vi "SMR_LabVIEW_V7.6.vi"() -> ()   [LabVIEW 2025]
uses:
  <vilib>/DAQmx/write.llb/DAQmx Write (Analog DBL 1Chan 1Samp).vi
  <vilib>/DAQmx/read.llb/DAQmx Read (Analog 1D DBL NChan 1Samp).vi
  <vilib>/DAQmx/read.llb/DAQmx Read (Analog 1D DBL 1Chan NSamp).vi
  <vilib>/Analysis/baseanly.llb/Mean (DBL).vi
  <vilib>/DAQmx/create/channels.llb/DAQmx Create Channel (AI-Temperature-Thermocouple).vi
  <vilib>/DAQmx/create/channels.llb/DAQmx Create Channel (AI-Voltage-Basic).vi
  <vilib>/DAQmx/create/channels.llb/DAQmx Create Channel (AO-Voltage-Basic).vi
  <vilib>/DAQmx/miscellaneous.llb/DAQmx Fill In Error Info.vi
  <vilib>/DAQmx/configure/timing.llb/DAQmx Timing (Sample Clock).vi
  <vilib>/addons/control/pid/pid.llb/PID (DBL).vi
  <vilib>/addons/control/pid/NI_PID_pid.lvlib
  <vilib>/Analysis/NI_AALBase.lvlib
panel:
  out "Voltage Across Rod (V)":dbl format="%0.2f"
  out "Current Run Folder":path
  in  "Log Root Folder":path=path "C:/Users/LocalUser/Documents/GitHub/thermal-loop/resources/v0.1.1/data/001"
  out "Raw NI9201 \nVoltage Display":T1
  in  "Loop Period (ms)":dbl=1000.0
  in  "Stop":bool
  out "Auto Steady State Threshold (deg C/min)":dbl
  out "Max dT/dt (deg C/min)":dbl
  out "Temp Change Rate (deg C/min)":dbl
  out "5-Min Baseline Complete":bool
  out "Rate Window Ready":bool
  out "Steady State":bool
  in  "Voltage Limit (V)":dbl=10.0
  in  "Temperature Limit (C)":dbl=50.0
  in  "Pressure Limit (psi)":dbl=15.0
  out "Max Voltage":bool
  out "Max Temperature":bool
  out "Max Pressure":bool
  out "Heat Exchanger Pressure History":dbl(graph)
  out "Main Loop Pressure History":T2(graph)
  out "Overall Avg Pressure (psi)":dbl
  out "Heat Exchanger Pressure P6 (psi)":dbl
  out "Main Loop Avg Pressure (psi)":dbl
  out "Pressure Display":T3
  out "Overall Pressure History":T4(graph)
  out "Max Loop Pressure (psi)":dbl
  out "Heat Exchanger Temperature History":cluster{"Waveform":dbl, "Waveform":dbl}(graph)
  out "Main Loop Temeperature History":T5(graph)
  out "Heat Exchanger Avg Temp (deg C)":dbl
  out "Temperature Display":T6
  out "Overall Temperature History":T7(graph)
  out "Overall Avg Temp (deg C)":dbl
  out "Max Loop Temp (deg C)":dbl
  out "Final P-Valve Voltage (V)":dbl
  out "PID Trim Voltage (V)":dbl
  in  "PID Temp Setpoint (deg C)":dbl
  in  "Auto PID Enable":bool
  in  "Manual P-Valve Voltage (V)":dbl min=0.0 max=10.0
  out "Main Loop Avg Temp (deg C)":dbl
  out "Flow History":dbl(graph)
  out "Heat Exchanger Flow (GPM)":dbl
  # "Control/Troubleshoot"
  # "Steady State"
  # "Emergency Indicators"
  # "Pressure"
  # "Temperature"
  # "Proportional Valve Control"
  # "Heat Exchanger Flow"
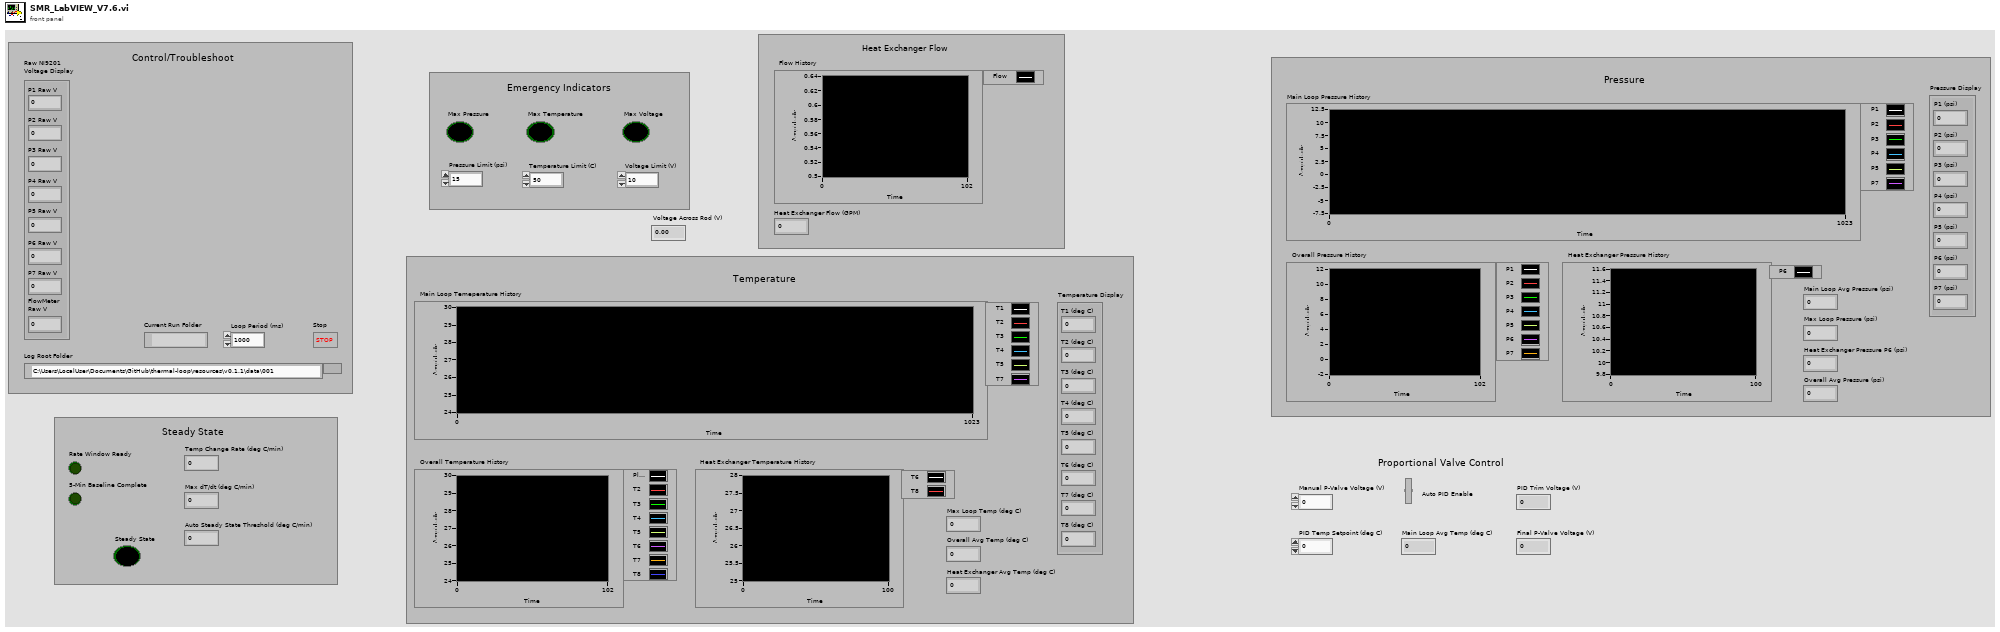
[diagram p1: front panel]
types:
  T1 = cluster{"P1 Raw V":dbl, "P2 Raw V":dbl, "P3 Raw V":dbl, "P4 Raw V":dbl, "P5 Raw V":dbl, "P6 Raw V":dbl, "P7 Raw V":dbl, "FlowMeter\nRaw V":dbl}
  T2 = cluster{"P1":dbl, "P2":dbl, "P3":dbl, "P4":dbl, "P5":dbl, "P7":dbl}
  T3 = cluster{"P1 (psi)":dbl, "P2 (psi)":dbl, "P3 (psi)":dbl, "P4 (psi)":dbl, "P5 (psi)":dbl, "P6 (psi)":dbl, "P7 (psi)":dbl}
  T4 = cluster{"P1":dbl, "P2":dbl, "P3":dbl, "P4":dbl, "P5":dbl, "P6":dbl, "P7":dbl}
  T5 = cluster{"Waveform":dbl, "Waveform":dbl, "Waveform":dbl, "Waveform":dbl, "Waveform":dbl, "Waveform":dbl}
  T6 = cluster{"T1 (deg C)":dbl, "T2 (deg C)":dbl, "T3 (deg C)":dbl, "T4 (deg C)":dbl, "T5 (deg C)":dbl, "T6 (deg C)":dbl, "T7 (deg C)":dbl, "T8 (deg C)":dbl}
  T7 = cluster{"Waveform":dbl, "Waveform":dbl, "Waveform":dbl, "Waveform":dbl, "Waveform":dbl, "Waveform":dbl, "Waveform":dbl, "Waveform":dbl}
  T8 = enum16{"open", "replace", "create", "open or create", "replace or create", "replace or create with confirmation"}
  T9 = cluster{"proportional gain (Kc)":dbl, "integral time (Ti, min)":dbl, "derivative time (Td, min)":dbl}
  T10 = cluster{"P1":dbl, "P2":dbl, "P3":dbl, "P4":dbl, "P5":dbl, "P6":dbl, "P7":dbl, "Flow":dbl}
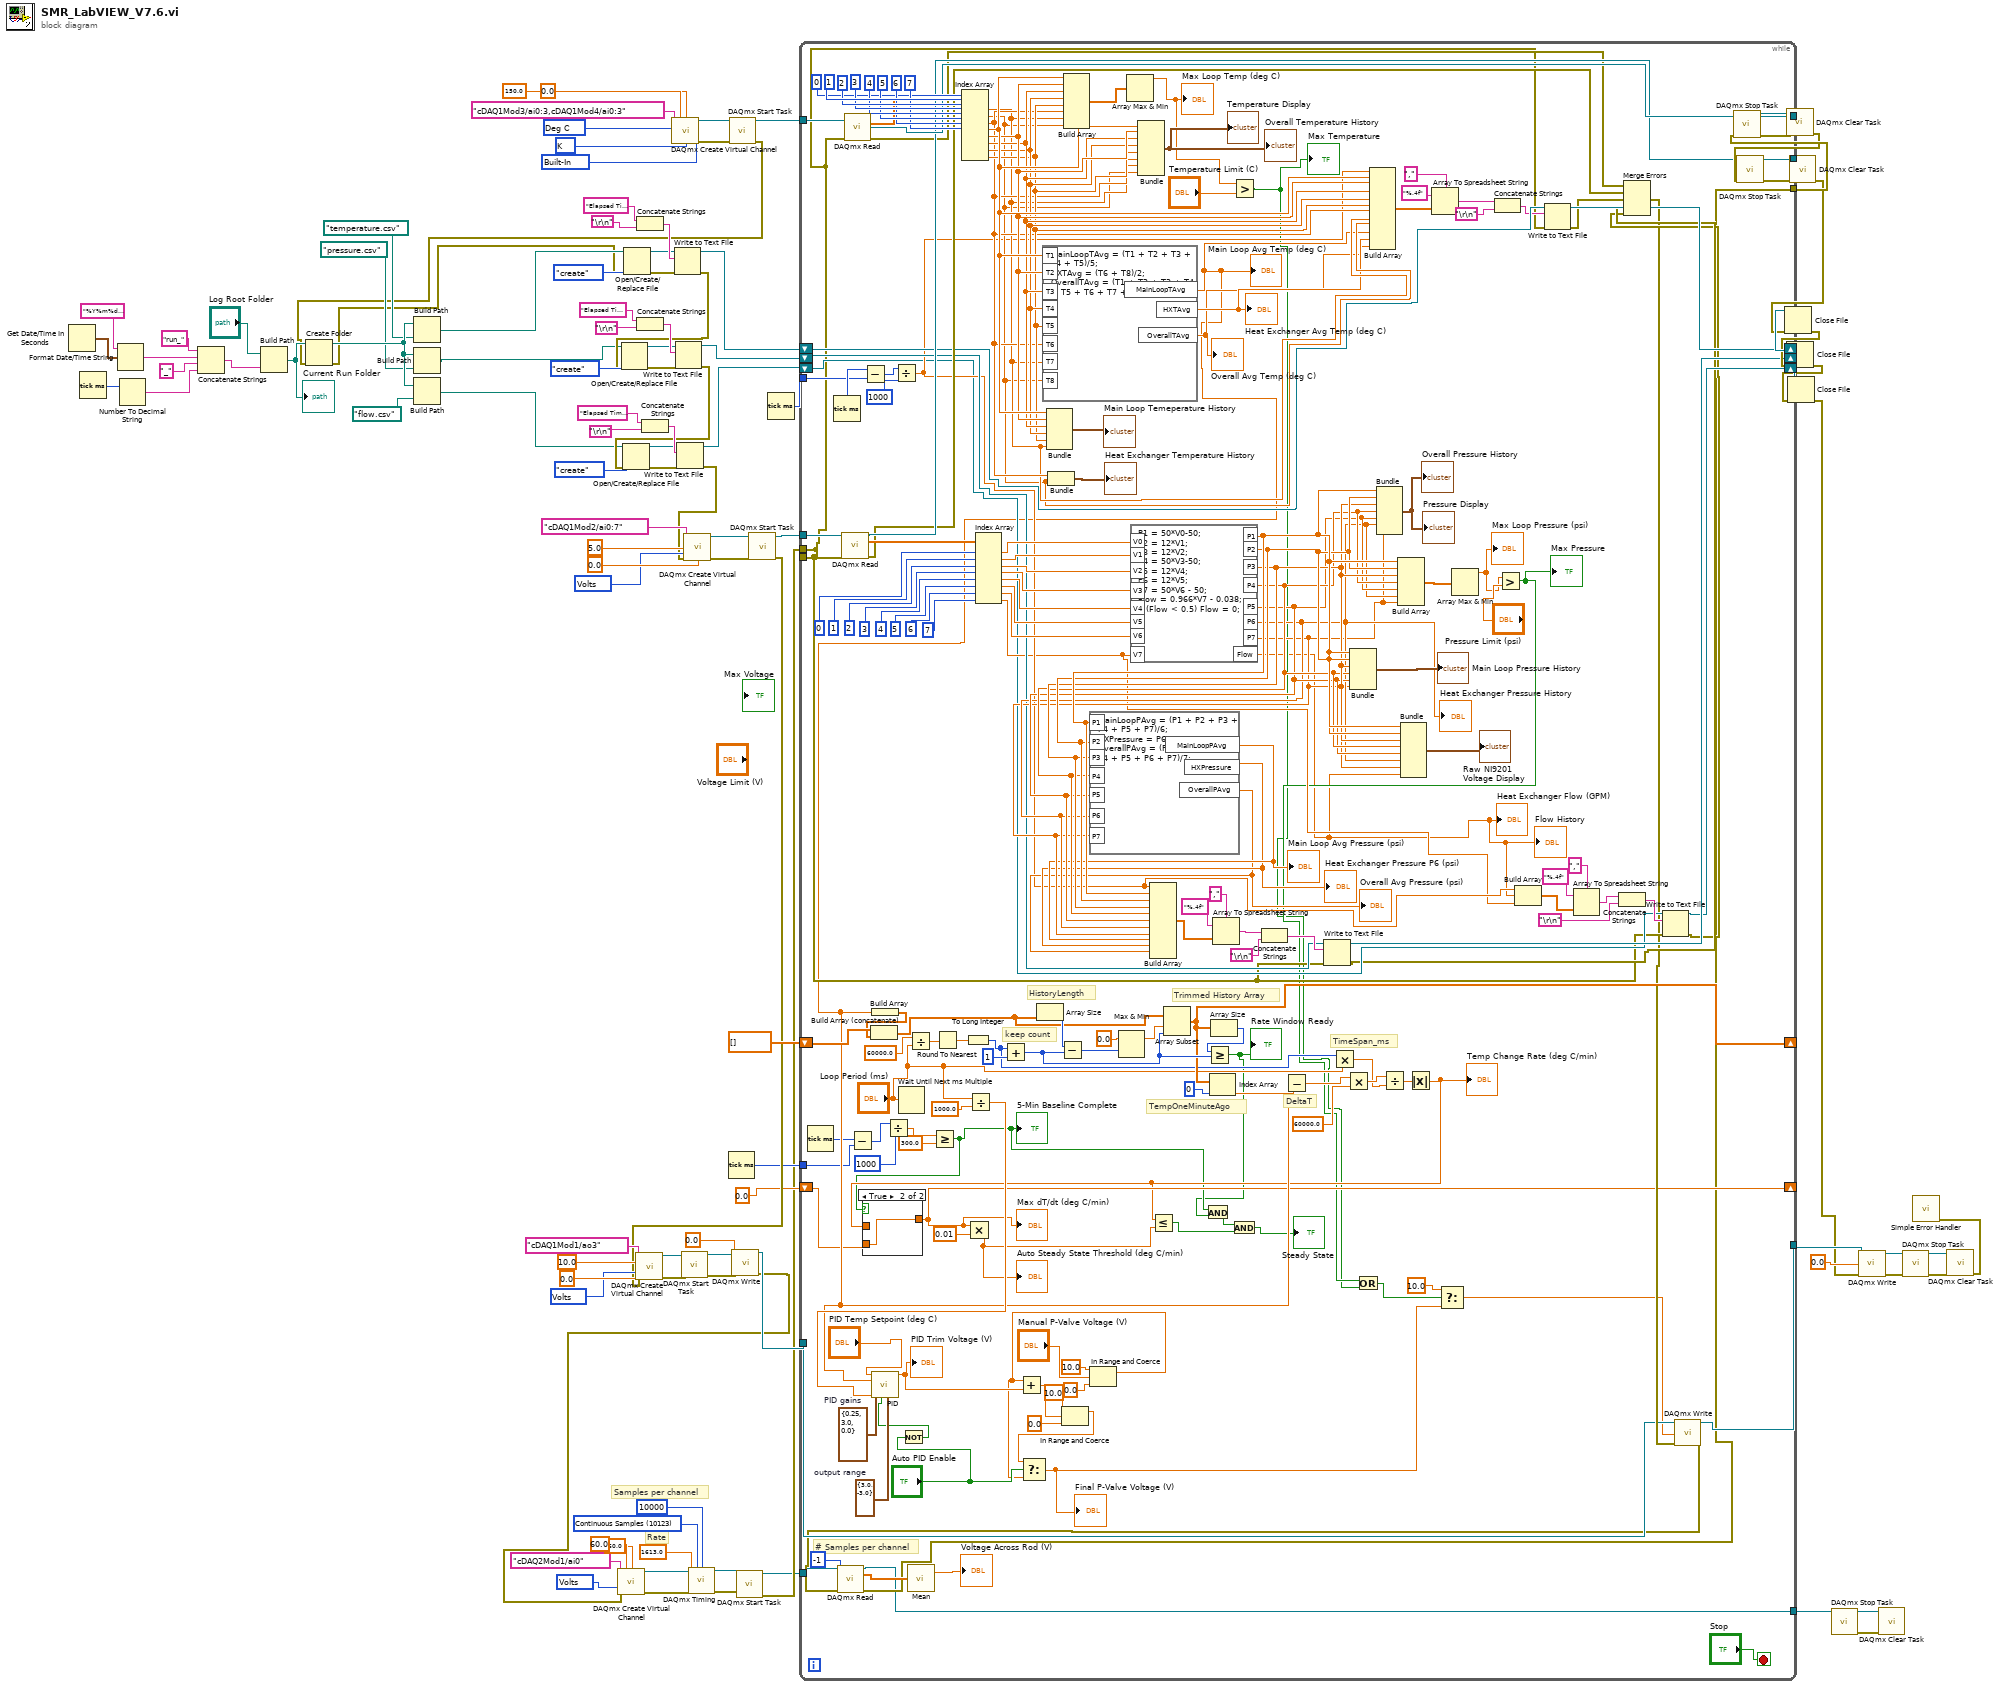
[diagram p0: block diagram]
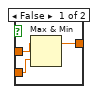
[diagram p2: hidden frame]
diagram:
  w12 = 10123 items=["Finite Samples"=10178, "Continuous Samples"=10123, "Hardware Timed Single Point"=12522] ("sample mode")
  w14 = 10348 items=["Volts"=10348, "From Custom Scale"=10065] ("units")
  w35 = 10348 items=["Volts"=10348, "From Custom Scale"=10065] ("units")
  w101 = 10200 items=["Built-In"=10200, "Constant Value"=10116, "Channel"=10113] ("cjc source")
  w102 = 10073 items=["J"=10072, "K"=10073, "N"=10077, "R"=10082, "S"=10085, "T"=10086, "B"=10047, "E"=10055] ("thermocouple type")
  w103 = 10143 items=["Deg C"=10143, "Deg F"=10144, "Kelvins"=10325, "Deg R"=10145, "From Custom Scale"=10065] ("units")
  w110 = 10348 items=["Volts"=10348, "From Custom Scale"=10065] ("units")
  # "Samples per channel"
  # "Rate"
  n1 = Get Date/Time In Seconds() -> (seconds since 1Jan1904=w58:timestamp)
  n2 = Tick Count (ms)() -> (millisecond timer value=w56:u32)
  n3 = Format Date/Time String(time format string (%c)="%Y%m%d_%H%M%S", seconds (now)=w58) -> (date/time string=w53:string)  [unwired: 1 in]
  n4 = Number To Decimal String(number=w56) -> (decimal integer string=w54:string)  [unwired: 1 in]
  n5 = Concatenate Strings("run_" ("string"), w53, "_" ("string"), w54) -> (w50:string)
  n6 = Build Path(base path="Log Root Folder", name or relative path=w50) -> (appended path=w49:path)
  "Current Run Folder" <- w49
  n7 = Concatenate Strings("Elapsed Time (s),T1 (deg C),T2 (deg C),T3 (deg C),T4 (deg C),T5 (deg C),T6 (deg C),T7 (deg C),T8 (deg C),Main Loop Avg Temp (deg C),HX Avg Temp (deg C),Overall Avg Temp (deg C)", "\r\n") -> (w84:string)
  n8 = Concatenate Strings("Elapsed Time (s),P1 (psi),P2 (psi),P3 (psi),P4 (psi),P5 (psi),P6 (psi),P7 (psi),Main Loop Avg Pressure (psi),HX Pressure (psi),Overall Avg Pressure (psi)", "\r\n") -> (w82:string)
  n9 = Concatenate Strings("Elapsed Time (s),Heat Exchanger Flow (GPM),Flow Raw Voltage (V)", "\r\n") -> (w78:string)
  n10 = call-poly <vilib>:"DAQmx Create Virtual Channel.vi"("maximum value"=150.0, "minimum value"=0.0, "physical channels"=tag "cDAQ1Mod3/ai0:3,cDAQ1Mod4/ai0:3", "cjc source"=w101, "units"=w103, "thermocouple type"=w102) -> ("task out"=w100:refnum<k21>, "error out"=w99:errorcluster)  [unwired: 8 in]
  n11 = Tick Count (ms)() -> (millisecond timer value=w19:u32)
  n12 = call <vilib>:"DAQmx Start Task.vi"("task/channels in"=w100, "error in"=w99) -> ("task out"=w98:refnum<k21>, "error out"=w41:errorcluster)  [unwired: 12 in]
  n13 = Create Folder(path (use dialog)=w49, error in=w41) -> (created path=w48:path, error out=w40:errorcluster)  [unwired: 1 in, 1 out]
  n14 = Build Path(base path=w48, name or relative path=path "temperature.csv") -> (appended path=w47:path)
  n15 = Build Path(base path=w48, name or relative path=path "pressure.csv") -> (appended path=w46:path)
  n16 = Build Path(base path=w48, name or relative path=path "flow.csv") -> (appended path=w45:path)
  n17 = Open/Create/Replace File(file path (use dialog)=w47, error in=w40, operation (0:open)=T8."create") -> (refnum out=w83:refnum<file>, error out=w67:errorcluster)  [unwired: 3 in, 1 out]
  n18 = Write to Text File(file (use dialog)=w83, text=w84, error in=w67) -> (refnum out=w74:refnum<file>, error out=w66:errorcluster)  [unwired: 1 in, 1 out]
  n19 = Open/Create/Replace File(file path (use dialog)=w46, error in=w66, operation (0:open)=T8."create") -> (refnum out=w81:refnum<file>, error out=w65:errorcluster)  [unwired: 3 in, 1 out]
  n20 = Write to Text File(file (use dialog)=w81, text=w82, error in=w65) -> (refnum out=w73:refnum<file>, error out=w64:errorcluster)  [unwired: 1 in, 1 out]
  n21 = Open/Create/Replace File(file path (use dialog)=w45, error in=w64, operation (0:open)=T8."create") -> (refnum out=w77:refnum<file>, error out=w63:errorcluster)  [unwired: 3 in, 1 out]
  n22 = Write to Text File(file (use dialog)=w77, text=w78, error in=w63) -> (refnum out=w72:refnum<file>, error out=w62:errorcluster)  [unwired: 1 in, 1 out]
  n23 = call-poly <vilib>:"DAQmx Create Virtual Channel.vi"("maximum value"=5.0, "minimum value"=0.0, "physical channels"=tag "cDAQ1Mod2/ai0:7", "units"=w110, "error in"=w62) -> ("task out"=w109:refnum<k21>, "error out"=w108:errorcluster)  [unwired: 9 in]
  n24 = call <vilib>:"DAQmx Start Task.vi"("task/channels in"=w109, "error in"=w108) -> ("task out"=w107:refnum<k21>, "error out"=w28:errorcluster)  [unwired: 12 in]
  n25 = call-poly <vilib>:"DAQmx Create Virtual Channel.vi"("maximum value"=10.0, "minimum value"=0.0, "physical channels"=tag "cDAQ1Mod1/ao3", "units"=w35, "error in"=w28) -> ("task out"=w34:refnum<k21>, "error out"=w33:errorcluster)  [unwired: 9 in]
  n26 = call <vilib>:"DAQmx Start Task.vi"("task/channels in"=w34, "error in"=w33) -> ("task out"=w32:refnum<k21>, "error out"=w31:errorcluster)  [unwired: 12 in]
  n27 = call-poly <vilib>:"DAQmx Write.vi"("task/channels in"=w32, "data"=0.0, "error in"=w31) -> ("task out"=w29:refnum<k21>, "error out"=w6:errorcluster)  [unwired: 10 in, 1 out]
  n28 = call-poly <vilib>:"DAQmx Create Virtual Channel.vi"("maximum value"=60.0, "minimum value"=-60.0, "physical channels"=tag "cDAQ2Mod1/ai0", "units"=w14, "error in"=w6) -> ("task out"=w3:refnum<k21>, "error out"=w5:errorcluster)  [unwired: 9 in]
  n29 = call-poly <vilib>:"DAQmx Timing.vi"("task/channels in"=w3, "sample mode"=w12, "samples per channel"=10000, "rate"=1613.0, "error in"=w5) -> ("task out"=w10:refnum<k21>, "error out"=w9:errorcluster)  [unwired: 9 in]
  n30 = call <vilib>:"DAQmx Start Task.vi"("task/channels in"=w10, "error in"=w9) -> ("task out"=w2:refnum<k21>, "error out"=w4:errorcluster)  [unwired: 12 in]
  n31 = Tick Count (ms)() -> (millisecond timer value=w71:u32)
  n32 = while {
    tunnel: w107 -> [w282]
    tunnel: w98 -> [w258]
    tunnel: [w248] -> w97
    tunnel: [w163] -> _
    tunnel: [w247] -> w96
    tunnel: [w117] -> w95
    shift-right: [w224] -> w70
    shift-left: w74 -> [w225]
    shift-right: [w205] -> w69
    shift-left: w73 -> [w206]
    shift-right: [w195] -> w68
    shift-left: w72 -> [w196]
    tunnel: w71 -> [w243]
    shift-right: [w174] -> _
    shift-left: dbl[] [] -> [w187]
    tunnel: w29 -> [w154]
    tunnel: w4 -> [w163]
    tunnel: [w161] -> w26
    tunnel: w19 -> [w143]
    shift-right: [w136] -> _
    shift-left: 0.0 -> [w138]
    tunnel: w2 -> [w116]
    tunnel: [w115] -> w1
    stop <- "Stop" stop-if-true
    w159 = cluster{"output high":dbl, "output low":dbl} {"output high"=3.0, "output low"=-3.0}  # output range
    w160 = T9 {"proportional gain (Kc)"=0.25, "integral time (Ti, min)"=3.0, "derivative time (Td, min)"=0.0}  # PID gains
    # "# Samples per channel"
    # "TimeSpan_ms"
    # "DeltaT"
    # "TempOneMinuteAgo"
    # "Trimmed History Array"
    # "HistoryLength"
    # "keep count"
    n33 = Tick Count (ms)() -> (millisecond timer value=w144:u32)
    n34 = Tick Count (ms)() -> (millisecond timer value=w244:u32)
    n35 = call-poly <vilib>:"DAQmx Read.vi"("task/channels in"=w282, "error in"=w163) -> ("task out"=w247:refnum<k21>, "data"=w273:dbl[], "error out"=w245:errorcluster)  [unwired: 11 in]
    n36 = call-poly <vilib>:"DAQmx Read.vi"("task/channels in"=w258, "error in"=w163) -> ("task out"=w248:refnum<k21>, "data"=w249:dbl[], "error out"=w246:errorcluster)  [unwired: 11 in]
    n37 = Subtract(x=w144, y=w143) -> (x-y=w142:u32)
    n38 = Subtract(x=w244, y=w243) -> (x-y=w242:u32)
    n39 = Divide(x=w142, y=u32 1000) -> (x/y=w140:dbl)
    n40 = Divide(x=w242, y=u32 1000) -> (x/y=w204:dbl)
    n41 = Wait Until Next ms Multiple(millisecond multiple="Loop Period (ms)") -> ()  [unwired: 1 out]
    n42 = Not(x="Auto PID Enable") -> (.not. x?=w155:bool)
    n43 = Divide(x=60000.0, y="Loop Period (ms)") -> (x/y=w184:dbl)
    n44 = Greater Or Equal?(x=w140, y=300.0) -> (x >= y?=w133:bool)
    "5-Min Baseline Complete" <- w133
    n45 = Round To Nearest(number=w184) -> (nearest integer value=w183:dbl)
    n46 = Index Array(array=w249, index #1=0 ("index"), index #2=1 ("index"), index #3=2 ("index"), index #4=3 ("index"), index #5=4 ("index"), index #6=5 ("index"), index #7=6 ("index"), index #8=7 ("index")) -> (element #1=w234:dbl, element #2=w233:dbl, element #3=w235:dbl, element #4=w240:dbl, element #5=w239:dbl, element #6=w238:dbl, element #7=w237:dbl, element #8=w236:dbl)
    n47 = To Long Integer(number=w183) -> (32bit integer=w171:i32)
    n48 = Divide(x="Loop Period (ms)", y=1000.0) -> (x/y=w156:dbl)
    n49 = Index Array(array=w273, index #1=0 ("index"), index #2=1 ("index"), index #3=2 ("index"), index #4=3 ("index"), index #5=4 ("index"), index #6=5 ("index"), index #7=6 ("index"), index #8=7 ("index")) -> (element #1=w272:dbl, element #2=w271:dbl, element #3=w270:dbl, element #4=w269:dbl, element #5=w268:dbl, element #6=w267:dbl, element #7=w266:dbl, element #8=w203:dbl)
    n50 = Add(x=w171, y=1) -> (x+y=w176:i32)
    n51 = formula code="MainLoopTAvg = (T1 + T2 + T3 + T4 + T5)/5;\nHXTAvg = (T6 + T8)/2;\nOverallTAvg = (T1 + T2 + T3 + T4 + T5 + T6 + T7 + T8)/8;"("T1"=w240, "T2"=w239, "T3"=w238, "T4"=w237, "T5"=w236, "T6"=w235, "T7"=w234, "T8"=w233) -> ("MainLoopTAvg"=w146:dbl, "HXTAvg"=w232:dbl, "OverallTAvg"=w231:dbl)
    "Overall Avg Temp (deg C)" <- w231
    "Main Loop Avg Temp (deg C)" <- w146
    "Heat Exchanger Avg Temp (deg C)" <- w232
    n52 = Build Array(w146) -> (w186:dbl[])
    n53 = Build Array (concatenate)(w187, w186) -> (w178:dbl[])
    n54 = call-poly <vilib>:"PID.vi"("reinitialize? (F)"=w155, "output range"=w159, "dt (s)"=w156, "PID gains"=w160, "process variable"=w146, "setpoint"="PID Temp Setpoint (deg C)") -> ("output"=w153:dbl)  [unwired: 4 in, 1 out]
    "PID Trim Voltage (V)" <- w153
    n55 = Array Size(array=w178) -> (size(s)=w181:i32)
    n56 = Bundle("Waveform"=w240, "Waveform"=w239, "Waveform"=w238, "Waveform"=w237, "Waveform"=w236, "Waveform"=w234) -> (→"Main Loop Temeperature History":T5)  [unwired: 1 in]
    n57 = Bundle("Waveform"=w235, "Waveform"=w233) -> (→"Heat Exchanger Temperature History":cluster{"Waveform":dbl, "Waveform":dbl})  [unwired: 1 in]
    n58 = Subtract(x=w181, y=w176) -> (x-y=w179:i32)
    n59 = Build Array(w240, w239, w238, w237, w236, w235, w234, w233) -> (w283:dbl[])
    n60 = In Range and Coerce(upper limit=10.0, x="Manual P-Valve Voltage (V)", lower limit=0.0) -> (coerced(x)=w148:dbl)  [unwired: 1 out]
    n61 = Add(x=w148, y=w153) -> (x+y=w152:dbl)
    n62 = In Range and Coerce(upper limit=10.0, x=w152, lower limit=0.0) -> (coerced(x)=w147:dbl)  [unwired: 1 out]
    n63 = Select(t=w147, s="Auto PID Enable", f=w148) -> (s? t:f=w124:dbl)
    "Final P-Valve Voltage (V)" <- w124
    n64 = Max & Min(x=0.0, y=w179) -> (max(x,y)=w177:dbl)  [unwired: 1 out]
    n65 = Array Max & Min(array=w283) -> (max value=w189:dbl)  [unwired: 3 out]
    "Max Loop Temp (deg C)" <- w189
    n66 = formula code="P1 = 50*V0-50;\nP2 = 12*V1;\nP3 = 12*V2;\nP4 = 50*V3-50;\nP5 = 12*V4;\nP6 = 12*V5; \nP7 = 50*V6 - 50;\nFlow = 0.966*V7 - 0.038;\nif (Flow < 0.5) Flow = 0;"("V0"=w272, "V1"=w271, "V2"=w270, "V3"=w269, "V4"=w268, "V5"=w267, "V6"=w266, "V7"=w203) -> ("P1"=w223:dbl, "P2"=w222:dbl, "P3"=w221:dbl, "P4"=w220:dbl, "P5"=w219:dbl, "P6"=w218:dbl, "P7"=w217:dbl, "Flow"=w114:dbl)
    "Heat Exchanger Flow (GPM)" <- w114
    "Flow History" <- w114
    "Heat Exchanger Pressure History" <- w218
    n67 = formula code="MainLoopPAvg = (P1 + P2 + P3 + P4 + P5 + P7)/6;\nHXPressure = P6;\nOverallPAvg = (P1 + P2 + P3 + P4 + P5 + P6 + P7)/7;"("P1"=w223, "P2"=w222, "P3"=w221, "P4"=w220, "P5"=w219, "P6"=w218, "P7"=w217) -> ("MainLoopPAvg"=w216:dbl, "HXPressure"=w215:dbl, "OverallPAvg"=w214:dbl)
    "Overall Avg Pressure (psi)" <- w214
    "Heat Exchanger Pressure P6 (psi)" <- w215
    "Main Loop Avg Pressure (psi)" <- w216
    n68 = Bundle("Waveform"=w240, "Waveform"=w239, "Waveform"=w238, "Waveform"=w237, "Waveform"=w236, "Waveform"=w235, "Waveform"=w234, "Waveform"=w233) -> (→"Overall Temperature History" →"Temperature Display":T7)  [unwired: 1 in]
    n69 = Build Array(w204, w223, w222, w221, w220, w219, w218, w217, w216, w215, w214) -> (w213:dbl[])
    n70 = Array Subset(array=w178, index=w177, length=w176) -> (w174:dbl[])
    n71 = Index Array(array=w174, index=0) -> (element=w172:dbl)
    n72 = Array Size(array=w174) -> (size(s)=w175:i32)
    n73 = Greater Or Equal?(x=w175, y=w176) -> (x >= y?=w132:bool)
    "Rate Window Ready" <- w132
    n74 = And(x=w133, y=w132) -> (x .and. y?=w131:bool)
    n75 = Array To Spreadsheet String(delimiter (Tab)=",", array=w213, 3:"%.4f" ("format string")) -> (spreadsheet string=w209:string)
    n76 = Greater?(x=w189, y="Temperature Limit (C)") -> (0:w127:bool)
    "Max Temperature" <- w127
    n77 = Concatenate Strings(w209, "\r\n") -> (w207:string)
    n78 = Subtract(x=w146, y=w172) -> (x-y=w170:dbl)
    n79 = Write to Text File(file (use dialog)=w206, text=w207, error in=w163) -> (refnum out=w205:refnum<file>, error out=w193:errorcluster)  [unwired: 1 in, 1 out]
    n80 = Multiply(x=w171, y="Loop Period (ms)") -> (x*y=w167:dbl)
    n81 = Multiply(x=w170, y=60000.0) -> (x*y=w168:dbl)
    n82 = Bundle("P1"=w223, "P2"=w222, "P3"=w221, "P4"=w220, "P5"=w219, "P7"=w217) -> (→"Main Loop Pressure History":T2)  [unwired: 1 in]
    n83 = Build Array(w204, w240, w239, w238, w237, w236, w235, w234, w233, w146, w232, w231) -> (w230:dbl[])
    n84 = Bundle("P1"=w223, "P2"=w222, "P3"=w221, "P4"=w220, "P5"=w219, "P6"=w218, "P7"=w217) -> (→"Overall Pressure History" →"Pressure Display":T4)  [unwired: 1 in]
    n85 = Divide(x=w168, y=w167) -> (x/y=w166:dbl)
    n86 = Build Array(w223, w222, w221, w220, w219, w218, w217) -> (w265:dbl[])
    n87 = Bundle("P1"=w223, "P2"=w222, "P3"=w221, "P4"=w220, "P5"=w219, "P6"=w218, "P7"=w217, "Flow"=w114) -> (→"Raw NI9201 \nVoltage Display":T10)  [unwired: 1 in]
    n88 = Absolute Value(x=w166) -> (abs(x)=w135:dbl)
    "Temp Change Rate (deg C/min)" <- w135
    n89 = case shown="True" w133 {
      tunnel: w138 -> [w287 w288]
      tunnel: w135 -> [w286 _]
      tunnel: [w285 w288] -> w136
      frame False {
        n90 = Max & Min(x=w286, y=w287) -> (max(x,y)=w285:dbl)  [unwired: 1 out]
      }
      frame True {
      }
    }
    "Max dT/dt (deg C/min)" <- w136
    n91 = Multiply(x=w136, y=0.01) -> (x*y=w134:dbl)
    "Auto Steady State Threshold (deg C/min)" <- w134
    n92 = Less Or Equal?(x=w135, y=w134) -> (x <= y?=w130:bool)
    n93 = And(x=w131, y=w130) -> (x .and. y?=→"Steady State":bool)
    n94 = Array To Spreadsheet String(delimiter (Tab)=",", array=w230, 3:"%.4f" ("format string")) -> (spreadsheet string=w227:string)
    n95 = Array Max & Min(array=w265) -> (max value=w190:dbl)  [unwired: 3 out]
    "Max Loop Pressure (psi)" <- w190
    n96 = Concatenate Strings(w227, "\r\n") -> (w210:string)
    n97 = Greater?(x=w190, y="Pressure Limit (psi)") -> (0:w128:bool)
    "Max Pressure" <- w128
    n98 = Or(x=w128, y=w127) -> (x .or. y?=w122:bool)
    n99 = Select(t=10.0, s=w122, f=w124) -> (s? t:f=w123:dbl)
    n100 = Build Array(w204, w114, w203) -> (w202:dbl[])
    n101 = Write to Text File(file (use dialog)=w225, text=w210, error in=w163) -> (refnum out=w224:refnum<file>, error out=w194:errorcluster)  [unwired: 1 in, 1 out]
    n102 = Array To Spreadsheet String(delimiter (Tab)=",", array=w202, 3:"%.4f" ("format string")) -> (spreadsheet string=w198:string)
    n103 = Concatenate Strings(w198, "\r\n") -> (w197:string)
    n104 = Write to Text File(file (use dialog)=w196, text=w197, error in=w163) -> (refnum out=w195:refnum<file>, error out=w192:errorcluster)  [unwired: 1 in, 1 out]
    n105 = Merge Errors(w246, w245, w194, w193, w192) -> (w162:errorcluster)
    n106 = call-poly <vilib>:"DAQmx Write.vi"("task/channels in"=w154, "data"=w123, "error in"=w162) -> ("task out"=w161:refnum<k21>, "error out"=w118:errorcluster)  [unwired: 10 in, 1 out]
    n107 = call-poly <vilib>:"DAQmx Read.vi"("task/channels in"=w116, "number of samples per channel"=-1, "error in"=w118) -> ("task out"=w115:refnum<k21>, "data"=w120:dbl[], "error out"=w117:errorcluster)  [unwired: 10 in]
    n108 = call-poly <vilib>:"Mean.vi"("X"=w120) -> ("mean"=→"Voltage Across Rod (V)":dbl)  [unwired: 1 out]
  }
  n109 = call <vilib>:"DAQmx Stop Task.vi"("task/channels in"=w97, "error in"=w95) -> ("task out"=w94:refnum<k21>, "error out"=w92:errorcluster)  [unwired: 12 in]
  n110 = call <vilib>:"DAQmx Clear Task.vi"("task in"=w94, "error in"=w92) -> ("error out"=w91:errorcluster)  [unwired: 13 in]
  n111 = call <vilib>:"DAQmx Stop Task.vi"("task/channels in"=w96, "error in"=w91) -> ("task out"=w93:refnum<k21>, "error out"=w90:errorcluster)  [unwired: 12 in]
  n112 = call <vilib>:"DAQmx Clear Task.vi"("task in"=w93, "error in"=w90) -> ("error out"=w61:errorcluster)  [unwired: 13 in]
  n113 = Close File(refnum=w70, error in=w61) -> (error out=w60:errorcluster)  [unwired: 1 out]
  n114 = Close File(refnum=w69, error in=w60) -> (error out=w59:errorcluster)  [unwired: 1 out]
  n115 = Close File(refnum=w68, error in=w59) -> (error out=w25:errorcluster)  [unwired: 1 out]
  n116 = call <vilib>:"DAQmx Stop Task.vi"("task/channels in"=w1) -> ("task out"=w8:refnum<k21>, "error out"=w7:errorcluster)  [unwired: 13 in]
  n117 = call-poly <vilib>:"DAQmx Write.vi"("task/channels in"=w26, "data"=0.0, "error in"=w25) -> ("task out"=w24:refnum<k21>, "error out"=w22:errorcluster)  [unwired: 10 in, 1 out]
  n118 = call <vilib>:"DAQmx Clear Task.vi"("task in"=w8, "error in"=w7) -> ()  [unwired: 13 in, 1 out]
  n119 = call <vilib>:"DAQmx Stop Task.vi"("task/channels in"=w24, "error in"=w22) -> ("task out"=w23:refnum<k21>, "error out"=w21:errorcluster)  [unwired: 12 in]
  n120 = call <vilib>:"DAQmx Clear Task.vi"("task in"=w23, "error in"=w21) -> ("error out"=w20:errorcluster)  [unwired: 13 in]
  n121 = call <vilib>:"Simple Error Handler.vi"("error in (no error)"=w20) -> ()  [unwired: 4 in, 5 out]
